vi "Export Skipped.vi"(8 "error in (no error)":errorcluster, 10 "Message":string, 11 "Node in":refnum<k20>) -> (0 "error out":errorcluster, 3 "Node out":refnum<k20>)   [LabVIEW 2013, in "JUnit for Azure Pipelines.lvclass"]
uses:
  JUnit for Azure Pipelines.lvclass
  <vilib>/xml/Close Reference(Node).vi
  <vilib>/xml/NI_XML.lvlib
  XML/XML.lvlib
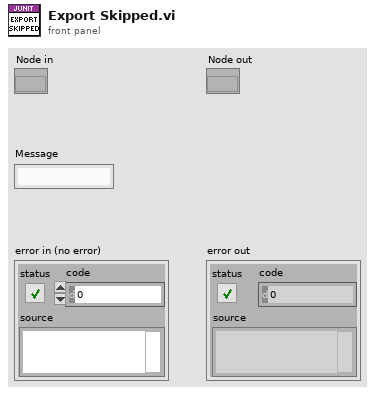
[diagram p1: front panel]
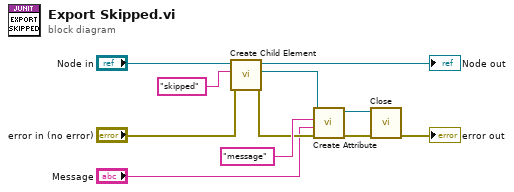
[diagram p0: block diagram]
diagram:
  n1 = call "Create Child Element.vi"("error in (no error)"="error in (no error)", "Name"="skipped" ("Tag Name"), "Element in"="Node in") -> ("error out"=w2:errorcluster, "Child Element"=w3:refnum<k20>, "Element out"=→"Node out":refnum<k20>)  [unwired: 6 in]
  n2 = call "Create Attribute.vi"("error in (no error)"=w2, "Value"="Message", "Name"="message" ("Attribute Name"), "Element in"=w3) -> ("error out"=w4:errorcluster, "Element out"=w5:refnum<k20>)  [unwired: 6 in]
  n3 = call-poly <vilib>:"Close.vi"("error in (no error)"=w4, "node"=w5) -> ("error out"=→"error out":errorcluster)  [unwired: 7 in]
